vi "FGV_Main.vi"() -> ()   [LabVIEW 2018]
panel:
  out "웨이브폼 차트 2":dbl(graph)
  out "웨이브폼 차트":dbl(graph)
  in  "정지 2":bool
  in  "정지":bool
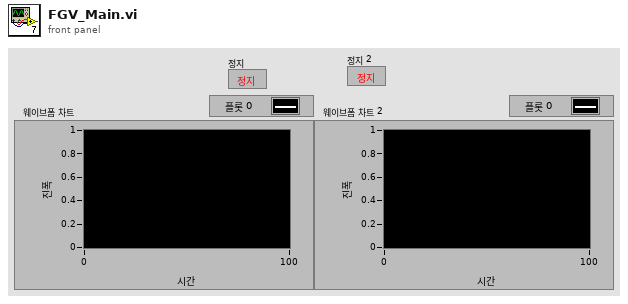
[diagram p1: front panel]
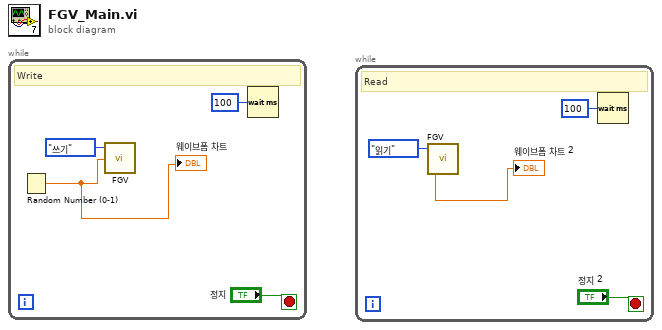
[diagram p0: block diagram]
diagram:
  n1 = while {
    stop <- "정지" stop-if-true
    # "Write"
    n2 = Random Number (0-1)() -> (number: 0 to 1=w1:dbl)
    "웨이브폼 차트" <- w1
    n3 = call "FGV.vi"("In"=w1, "상태 컨트롤"=enum16{"초기화", "읽기", "쓰기"}."쓰기") -> ()  [unwired: 1 in, 2 out]
    n4 = Wait (ms)(milliseconds to wait=u32 100 ("대기 시간 (ms)")) -> ()  [unwired: 1 out]
  }
  n5 = while {
    stop <- "정지 2" stop-if-true
    # "Read"
    n6 = call "FGV.vi"("상태 컨트롤"=enum16{"초기화", "읽기", "쓰기"}."읽기") -> ("Out"=→"웨이브폼 차트 2":dbl)  [unwired: 2 in, 1 out]
    n7 = Wait (ms)(milliseconds to wait=u32 100 ("대기 시간 (ms)")) -> ()  [unwired: 1 out]
  }
